vi "fgv_udp_srv-2.vi"(7 "cmd":enum16{"close", "rw", "ini"}(ring), 8 "error in":errorcluster caption="err-in", 11 "data_in":string) -> (0 "error out":errorcluster caption="err-out", 3 "data_out":string)   [LabVIEW 2017]
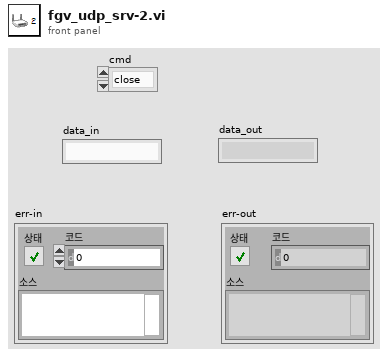
[diagram p1: front panel]
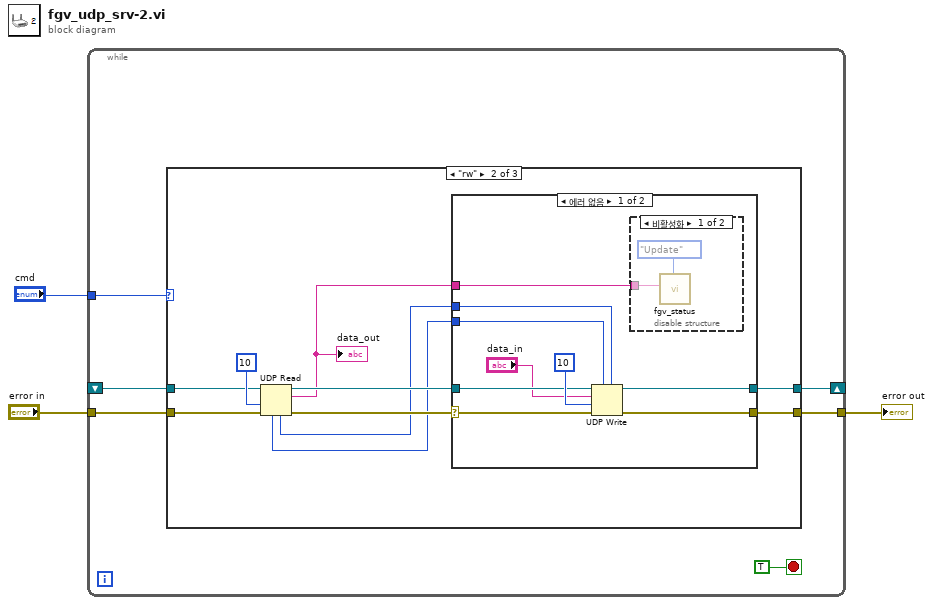
[diagram p0: block diagram]
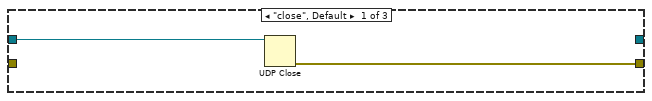
[diagram p2: hidden frame]
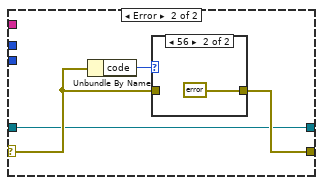
[diagram p4: hidden frame]
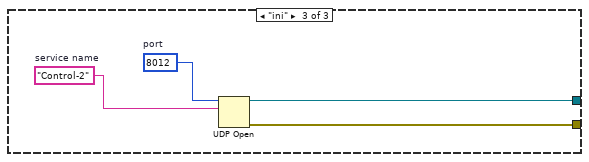
[diagram p6: hidden frame]
diagram:
  n1 = while {
    tunnel: "cmd" -> [w8]
    tunnel: "error in" -> [w7]
    tunnel: [w6] -> w1
    shift-right: [w5] -> _
    shift-left: _ -> [w4]
    stop <- TRUE stop-if-true
    n2 = case shown="\"rw\"" w8 {
      tunnel: w7 -> [_ w20 _]
      tunnel: [w10 w17 w40] -> w6
      tunnel: [_ w15 w39] -> w5
      tunnel: w4 -> [w11 w19 _]
      frame "close", Default {
        n3 = UDP Close(connection ID=w11) -> (error out=w10:errorcluster)  [unwired: 1 in, 1 out]
      }
      frame "rw" {
        n4 = UDP Read(connection ID=w19, timeout ms (25000)=10, 8:w20) -> (data out=w12:string, error out=w18:errorcluster, 3:w16:refnum<k16>, 4:w13:u16, 6:w14:u32)  [unwired: 1 in]
        "data_out" <- w12
        n5 = case shown="에러 없음" w18 {
          selector: w18 -> [w27 w34]
          tunnel: [w26 w35] -> w17
          tunnel: [w28 w33] -> w15
          tunnel: w16 -> [w29 w33]
          tunnel: w14 -> [w24 _]
          tunnel: w13 -> [w23 _]
          tunnel: w12 -> [w22 _]
          frame No Error {
            n6 = UDP Write(address=w24, port or service name=w23, connection ID=w29, data in="data_in", 8:w27, 9:10 ("타임아웃 ms (25000)")) -> (error out=w26:errorcluster, 3:w28:refnum<k16>)
            n7 = disable-structure shown="비활성화" {
              disable-tunnel: w22 -> [w31 _]
              frame Disabled {
                n8 = call "fgv_status.vi"("Mode"=enum16{"Initial", "Update", "Clear"}."Update", "String in"=w31) -> ()  [unwired: 9 in, 1 out]
              }
              frame Enabled {
              }
            }
          }
          frame Error {
            n9 = Unbundle By Name(w34) -> ("code"=w36:i32)
            n10 = case shown="56" w36 {
              tunnel: w34 -> [w37 _]
              tunnel: [w37 errorcluster {"status"=FALSE, "code"=0, "source"=""} ("No error")] -> w35
              frame Default {
              }
              frame 56 {
              }
            }
          }
        }
      }
      frame "ini" {
        w42 = u16 8012  # port
        w41 = "Control-2"  # service name
        n11 = UDP Open(10:w41, 11:w42) -> (port=w39:refnum<k16>, 0:w40:errorcluster)  [unwired: 3 in, 1 out]
      }
    }
  }
  "error out" <- w1
